vi "ALTS-2015 Robot Controller Loop.vi"(8 "error in (no error)":errorcluster) -> (0 "error out":errorcluster)   [LabVIEW 2013]
uses:
  Controls/ALTS-2015 Serial Details.ctl
  Controls/ALTS-2015 Robot Tasks.ctl
  Controls/ALTS-2015 Station Cluster.ctl
  Controls/ALTS-2015 Serial DB Details.ctl
  Robot Controller Queue/ALTS-2015 Robot Cotroller Options.ctl
  Controls/ALTS-2015 Auto Program States.ctl
  OPC Engine/Controls/ALTS-2015 OPC Read Registers.ctl
  OPC Engine/Controls/ALTS-2015 OPC Read Global Options.ctl
  Controls/ALTS-2015 Status Message Options.ctl
  Controls/ALTS-2015 Station Details.ctl
  Controls/ALTS-2015 Status Ring Indicator.ctl
  Controls/ALTS-2015 Robot Actions.ctl
  Controls/ALTS-2015 LV2GBL Station Info Options.ctl
  Controls/ALTS-2015 Robot FIFO Queue Options.ctl
  OPC Engine/Controls/ALTS-2015 OPC Write Registers.ctl
  OPC Engine/Controls/ALTS-2015 OPC Write Global Options.ctl
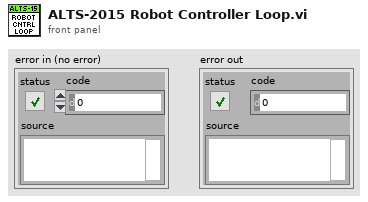
[diagram p1: front panel]
types:
  T1 = typedef "ALTS-2015 Robot Cotroller Options.ctl" = enum16{"Init", "Enqueue State", "Enqueue State in Opposite End", "Dequeue State", "Exit"}
  T2 = typedef "ALTS-2015 Auto Program States.ctl" = enum16{"<------ Robot Handler States ------>", "Wait for Robot Availability", "Check Last Task by Robot", "Wait & Read Task from Queue", "Write New Task Details to Robot", "Write Task Available for Robot", "Check Robot for Unavailbilty", "Write Task Unavailable for Robot", "<------------ Other ------------>", "Error", "Exit"}
  T3 = typedef "ALTS-2015 Serial Details.ctl" = cluster{"Robot Task":T4, "Serial No":string, "New Serial?":bool, "Station # Unload":T5, "Last Test Result":bool, "Rerun?":bool, "Station # Rerun":T5, "Invalid Serial?":bool, "Serial Details":T6}
  T4 = typedef "ALTS-2015 Robot Tasks.ctl" = enum16{"Load", "Unload", "Rerun", "Invalid Serial"}
  T5 = typedef "ALTS-2015 Station Cluster.ctl" = enum16{"Station 1", "Station 2", "Station 3", "Station 4"}
  T6 = typedef "ALTS-2015 Serial DB Details.ctl" = cluster{"Adapter Plate Size":i32, "Air Leak Test Type ":i32, "Displacement Size":i32, "Flange Size":i32, "Height":i32, "Load Decision":i32, "Cart Insert":i32}
  T7 = cluster{"Serial Details":T3, "Last Robot Task":T4, "Last Robot Task Out Station #":T5, "Robot Task broadcased?":bool}
  T8 = typedef "ALTS-2015 OPC Read Global Options.ctl" = enum16{"Init", "Write Value", "Write Array", "Read Value", "Read Array", "Read All"}
  T9 = typedef "ALTS-2015 OPC Read Registers.ctl" = enum16{"Robot_Available", "Start_Test", "Stop_Test", "Scan_Trigger", "Station_No_Start_Stop_Test"}
  T10 = typedef "ALTS-2015 Status Message Options.ctl" = enum16{"Initializing...", "Enter User Login...", "Valid Serial Number...", "Invalid Serial Number...", "Start Tag Received...", "Stop Tag Received...", "UUT Clamped...", "UUT not Clamped...", "Test Running...", "Test Complete...", "Task is assigned to robot...", "Robot is working on the task...", "Robot is ready for next task...", "Writing Result to DB...", "Idle...", "Exiting..."}
  T11 = typedef "ALTS-2015 LV2GBL Station Info Options.ctl" = enum16{"Init", "Read", "Read All", "Write Sensor ID", "Write  Work Order", "Write Serial Number", "Write Test Data", "Write Station Status", "Write Station Occupancy", "Write Station Test Type", "Write Rerun", "Write Load Decision", "Write Robot Action", "Clear All", "Clear Test Result"}
  T12 = typedef "ALTS-2015 Robot Actions.ctl" = enum16{"Loading...", "Unloading...", "Reruning...", "No Action"}
  T13 = typedef "ALTS-2015 Station Details.ctl" = cluster{"Station Number":string, "Work Order Number":string, "Sensor Name":string, "Pressure (PSI)":string, "Flow (SCCM)":string, "Test Time ":string, "Test Result":string, "Serial Number":string, "Station Status":T14, "SW assigned UUT":bool, "Rerun Count":i32, "Test Type":i32, "Load Decision":i32, "Robot Action":T12}
  T14 = typedef "ALTS-2015 Status Ring Indicator.ctl" = u16
  T15 = typedef "ALTS-2015 Robot FIFO Queue Options.ctl" = enum16{"Init", "Enqueue", "Dequeue", "Get Queue Elements", "Flush", "Destroy"}
  T16 = typedef "ALTS-2015 OPC Write Global Options.ctl" = enum16{"Init", "Write Value", "Write Array", "Read Value", "Read Array", "Read All"}
  T17 = typedef "ALTS-2015 OPC Write Registers.ctl" = enum16{"Task_Available_for_Robot", "New_Serial", "Serial_Adapter_Size", "Serial_Displacement_Size", "Serial_Flange_Size", "Serial_Height", "Serial_LoadDecision", "Serial_CartInsert", "Test_Result", "Station_Number", "Rerun", "Invalid_SNo", "PC_ACK_Read_Tags"}
  T18 = enum16{"Init", "Set - DB Loop", "Set - Robot Loop", "Get"}
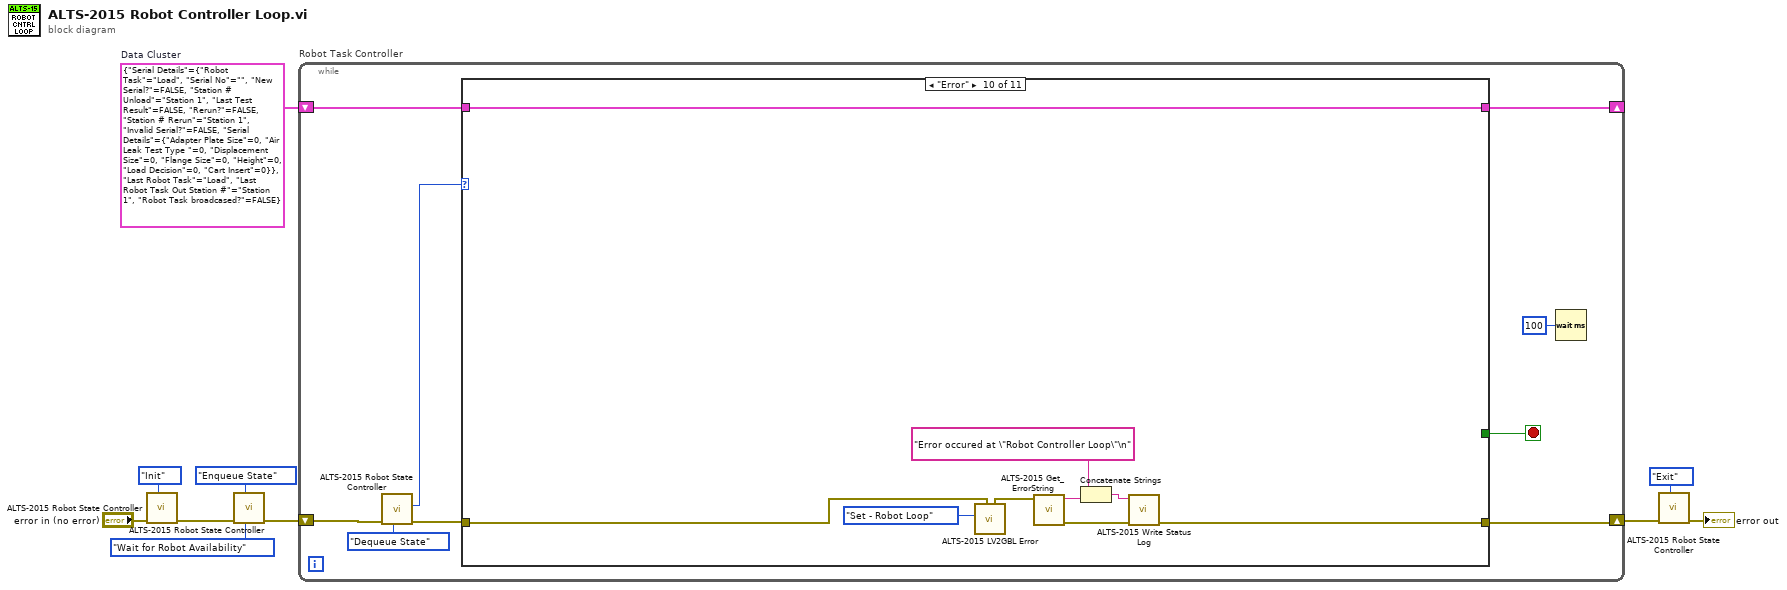
[diagram p0: block diagram]
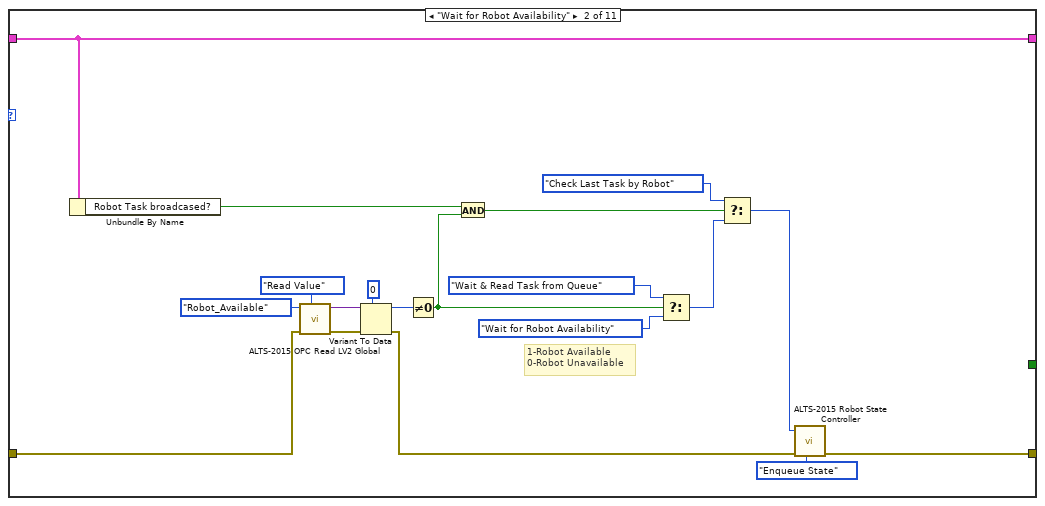
[diagram p3: hidden frame]
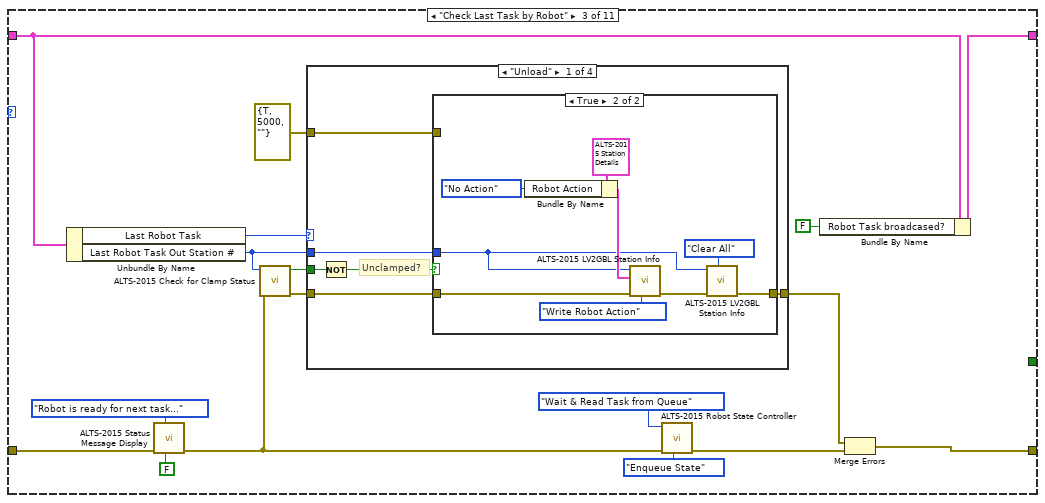
[diagram p4: hidden frame]
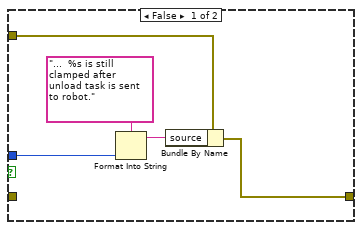
[diagram p5: hidden frame]
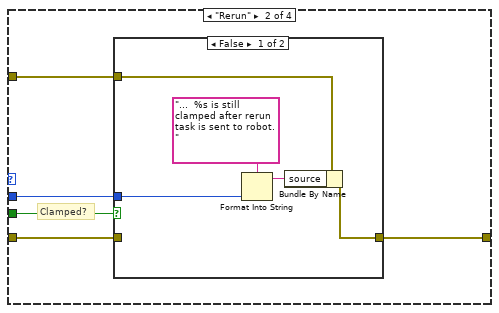
[diagram p6: hidden frame]
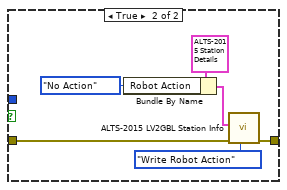
[diagram p7: hidden frame]
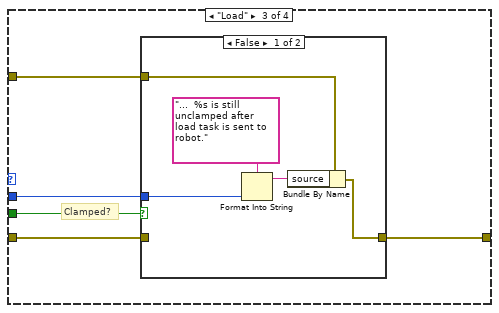
[diagram p8: hidden frame]
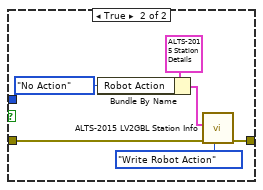
[diagram p9: hidden frame]
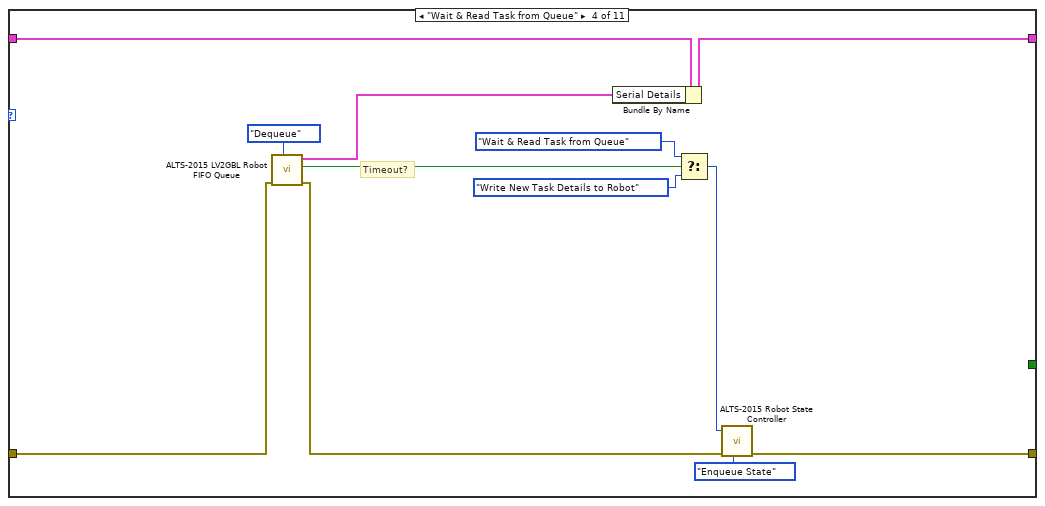
[diagram p11: hidden frame]
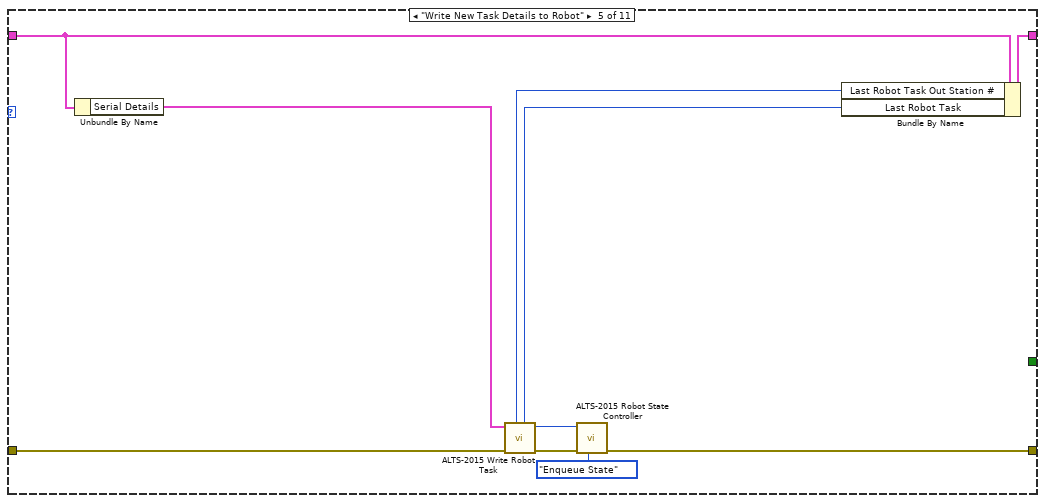
[diagram p12: hidden frame]
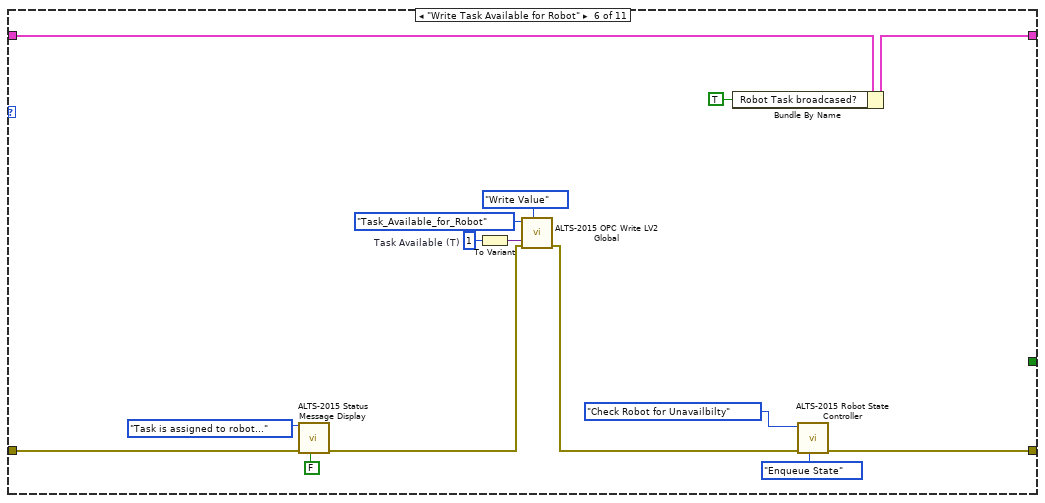
[diagram p13: hidden frame]
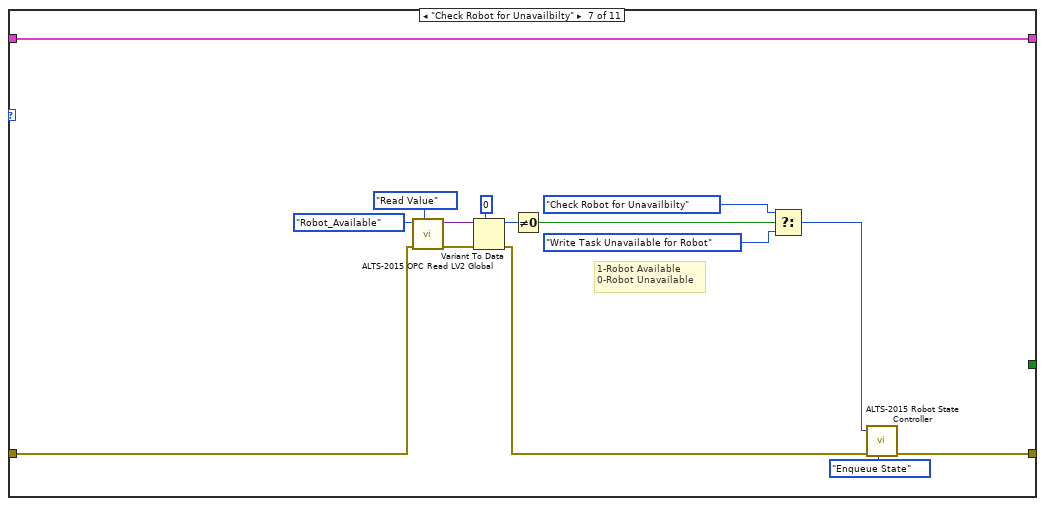
[diagram p14: hidden frame]
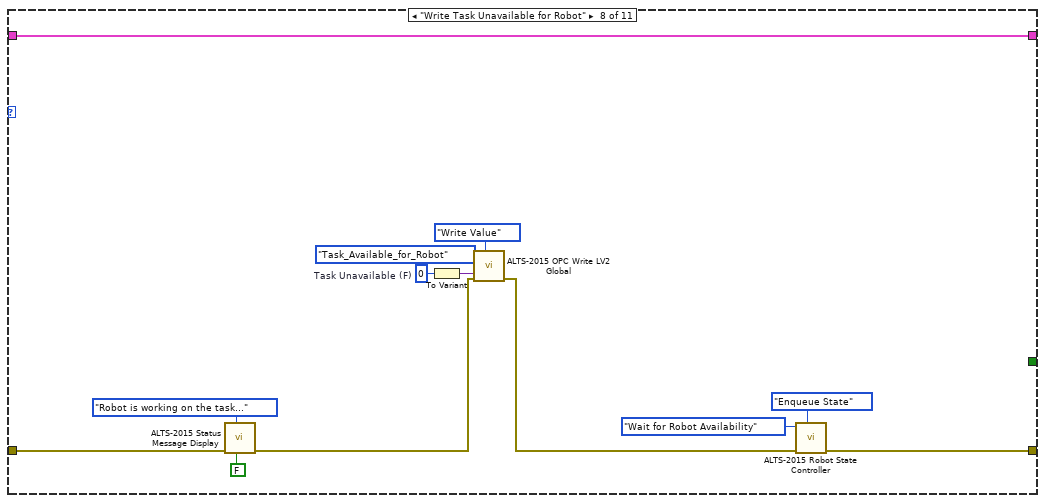
[diagram p15: hidden frame]
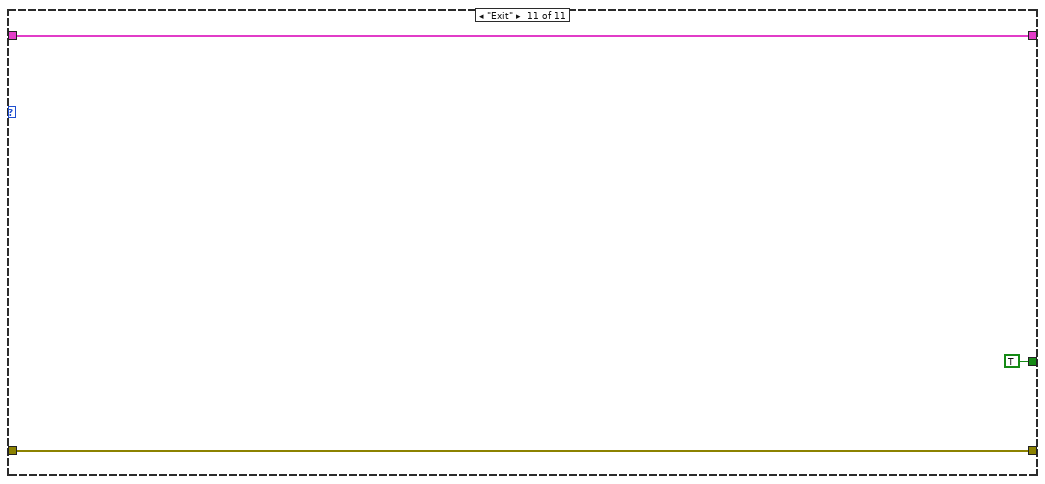
[diagram p17: hidden frame]
diagram:
  w9 = T7 {"Serial Details"={"Robot Task"=enum."Load", "Serial No"="", "New Serial?"=FALSE, "Station # Unload"=enum."Station 1", "Last Test Result"=FALSE, "Rerun?"=FALSE, "Station # Rerun"=enum."Station 1", "Invalid Serial?"=FALSE, "Serial Details"={"Adapter Plate Size"=0, "Air Leak Test Type "=0, "Displacement Size"=0, "Flange Size"=0, "Height"=0, "Load Decision"=0, "Cart Insert"=0}}, "Last Robot Task"=enum."Load", "Last Robot Task Out Station #"=enum."Station 1", "Robot Task broadcased?"=FALSE}  # Data Cluster
  n1 = call "ALTS-2015 Robot State Controller.vi"("Option"=ALTS-2015_Robot_Cotroller_Options."Init", "error in"="error in (no error)") -> ("error out"=w7:errorcluster)  [unwired: 8 in, 1 out]
  n2 = call "ALTS-2015 Robot State Controller.vi"("Option"=ALTS-2015_Robot_Cotroller_Options."Enqueue State", "error in"=w7, "Enqueue State"=ALTS-2015_Auto_Program_States."Wait for Robot Availability") -> ("error out"=w5:errorcluster)  [unwired: 7 in, 1 out]
  n3 = while "Robot Task Controller" {
    shift-right: [w11] -> w10
    shift-left: w5 -> [w15]
    shift-right: [w17] -> _
    shift-left: w9 -> [w18]
    stop <- w16 stop-if-true
    n4 = call "ALTS-2015 Robot State Controller.vi"("Option"=ALTS-2015_Robot_Cotroller_Options."Dequeue State", "error in"=w15) -> ("error out"=w14:errorcluster, "Dequeued State"=w13:T2)  [unwired: 8 in]
    n5 = case shown="\"Error\"" w13 {
      tunnel: [w20 w30 w43 w113 w128 w141 w150 w169 w176 w185 w188] -> w11
      tunnel: w14 -> [w20 w32 w44 w118 w132 w135 w156 w164 w176 w179 w188]
      tunnel: w18 -> [w21 w27 w55 w117 w131 w143 w153 w171 w177 w186 w189]
      tunnel: [w21 w27 w50 w116 w125 w138 w153 w171 w177 w186 w189] -> w17
      tunnel: [_ _ _ _ _ _ _ _ _ _ TRUE] -> w16
      frame "<------ Robot Handler States ------>" {
      }
      frame "Wait for Robot Availability" {
        # "1-Robot Available\n0-Robot Unavailable"
        n6 = Unbundle By Name(w27) -> ("Robot Task broadcased?"=w25:bool)
        n7 = call "ALTS-2015 OPC Read LV2 Global.vi"("Options"=ALTS-2015_OPC_Read_Global_Options."Read Value", "error in (no error)"=w32, "OPC Read Register"=ALTS-2015_OPC_Read_Registers."Robot_Available") -> ("error out"=w38:errorcluster, "OPC Read Reigter Value"=w39:variant)  [unwired: 6 in, 1 out]
        n8 = Variant To Data(error in=w38, type=0, Variant=w39) -> (data=w35:i32, error out=w31:errorcluster)
        n9 = Not Equal To 0?(x=w35) -> (x != 0?=w22:bool)
        n10 = And(x=w25, y=w22) -> (x .and. y?=w23:bool)
        n11 = Select(t=ALTS-2015_Auto_Program_States."Wait & Read Task from Queue", s=w22, f=ALTS-2015_Auto_Program_States."Wait for Robot Availability") -> (s? t:f=w29:T2)
        n12 = Select(t=ALTS-2015_Auto_Program_States."Check Last Task by Robot", s=w23, f=w29) -> (s? t:f=w26:T2)
        n13 = call "ALTS-2015 Robot State Controller.vi"("Option"=ALTS-2015_Robot_Cotroller_Options."Enqueue State", "error in"=w31, "Enqueue State"=w26) -> ("error out"=w30:errorcluster)  [unwired: 7 in, 1 out]
      }
      frame "Check Last Task by Robot" {
        n14 = Unbundle By Name(w55) -> ("Last Robot Task"=w51:T4, "Last Robot Task Out Station #"=w54:T5)
        n15 = call "ALTS-2015 Status Message Display.vi"("Station Message?"=FALSE, "Status Message Options"=ALTS-2015_Status_Message_Options."Robot is ready for next task...", "error in (no error)"=w44) -> ("error out"=w41:errorcluster)  [unwired: 7 in, 1 out]
        n16 = call "ALTS-2015 Check for Clamp Status .vi"("error in (no error)"=w41, "Station Cluster"=w54) -> ("error out"=w53:errorcluster, "Clamp?"=w52:bool)  [unwired: 8 in]
        n17 = case shown="\"Unload\"" w51 {
          tunnel: w54 -> [w63 w82 w98 _]
          tunnel: [w62 w81 w97 w110] -> w42
          tunnel: w53 -> [w61 w80 w96 w110]
          tunnel: w52 -> [w60 w79 w95 _]
          tunnel: errorcluster {"status"=TRUE, "code"=5000, "source"=""} ("error constant") -> [w58 w78 w94 _]
          frame "Unload" {
            # "Unclamped?"
            n18 = Not(x=w60) -> (.not. x?=w59:bool)
            n19 = case shown="True" w59 {
              tunnel: w63 -> [w68 w69]
              tunnel: w61 -> [_ w77]
              tunnel: [w66 w70] -> w62
              tunnel: w58 -> [w67 _]
              frame False {
                n20 = Format Into String(format string="...  %s is still clamped after unload task is sent to robot." ("Status Input"), w68) -> (resulting string=w64:string)  [unwired: 2 in, 1 out]
                n21 = Bundle By Name(cluster=w67, "source"=w64) -> (w66:errorcluster)
              }
              frame True {
                n22 = Bundle By Name(cluster=T13 {"Station Number"="", "Work Order Number"="", "Sensor Name"="", "Pressure (PSI)"="", "Flow (SCCM)"="", "Test Time "="", "Test Result"="", "Serial Number"="", "Station Status"=0, "SW assigned UUT"=FALSE, "Rerun Count"=0, "Test Type"=0, "Load Decision"=0, "Robot Action"=enum."Loading..."} ("Station"), "Robot Action"=ALTS-2015_Robot_Actions."No Action") -> (w75:T13)
                n23 = call "ALTS-2015 LV2GBL Station Info.vi"("Options"=ALTS-2015_LV2GBL_Station_Info_Options."Write Robot Action", "error in"=w77, "Station"=w75, "Station Cluster"=w69) -> ("error out"=w71:errorcluster)  [unwired: 5 in, 2 out]
                n24 = call "ALTS-2015 LV2GBL Station Info.vi"("Options"=ALTS-2015_LV2GBL_Station_Info_Options."Clear All", "error in"=w71, "Station Cluster"=w69) -> ("error out"=w70:errorcluster)  [unwired: 6 in, 2 out]
              }
            }
          }
          frame "Rerun" {
            # "Clamped?"
            n25 = case shown="False" w79 {
              tunnel: w82 -> [w87 _]
              tunnel: w80 -> [_ w90]
              tunnel: [w86 w89] -> w81
              tunnel: w78 -> [w84 _]
              frame False {
                n26 = Format Into String(format string="...  %s is still clamped after rerun task is sent to robot." ("Status Input"), w87) -> (resulting string=w83:string)  [unwired: 2 in, 1 out]
                n27 = Bundle By Name(cluster=w84, "source"=w83) -> (w86:errorcluster)
              }
              frame True {
                n28 = Bundle By Name(cluster=T13 {"Station Number"="", "Work Order Number"="", "Sensor Name"="", "Pressure (PSI)"="", "Flow (SCCM)"="", "Test Time "="", "Test Result"="", "Serial Number"="", "Station Status"=0, "SW assigned UUT"=FALSE, "Rerun Count"=0, "Test Type"=0, "Load Decision"=0, "Robot Action"=enum."Loading..."} ("Station"), "Robot Action"=ALTS-2015_Robot_Actions."No Action") -> (w92:T13)
                n29 = call "ALTS-2015 LV2GBL Station Info.vi"("Options"=ALTS-2015_LV2GBL_Station_Info_Options."Write Robot Action", "error in"=w90, "Station"=w92) -> ("error out"=w89:errorcluster)  [unwired: 6 in, 2 out]
              }
            }
          }
          frame "Load" {
            # "Clamped?"
            n30 = case shown="False" w95 {
              tunnel: w98 -> [w103 _]
              tunnel: w96 -> [_ w106]
              tunnel: [w100 w105] -> w97
              tunnel: w94 -> [w102 _]
              frame False {
                n31 = Format Into String(format string="...  %s is still unclamped after load task is sent to robot." ("Status Input"), w103) -> (resulting string=w99:string)  [unwired: 2 in, 1 out]
                n32 = Bundle By Name(cluster=w102, "source"=w99) -> (w100:errorcluster)
              }
              frame True {
                n33 = Bundle By Name(cluster=T13 {"Station Number"="", "Work Order Number"="", "Sensor Name"="", "Pressure (PSI)"="", "Flow (SCCM)"="", "Test Time "="", "Test Result"="", "Serial Number"="", "Station Status"=0, "SW assigned UUT"=FALSE, "Rerun Count"=0, "Test Type"=0, "Load Decision"=0, "Robot Action"=enum."Loading..."} ("Station"), "Robot Action"=ALTS-2015_Robot_Actions."No Action") -> (w108:T13)
                n34 = call "ALTS-2015 LV2GBL Station Info.vi"("Options"=ALTS-2015_LV2GBL_Station_Info_Options."Write Robot Action", "error in"=w106, "Station"=w108) -> ("error out"=w105:errorcluster)  [unwired: 6 in, 2 out]
              }
            }
          }
          frame Default {
          }
        }
        n35 = call "ALTS-2015 Robot State Controller.vi"("Option"=ALTS-2015_Robot_Cotroller_Options."Enqueue State", "error in"=w41, "Enqueue State"=ALTS-2015_Auto_Program_States."Wait & Read Task from Queue") -> ("error out"=w57:errorcluster)  [unwired: 7 in, 1 out]
        n36 = Bundle By Name(cluster=w55, "Robot Task broadcased?"=FALSE) -> (w50:T7)
        n37 = Merge Errors(w42, w57) -> (w43:errorcluster)
      }
      frame "Wait & Read Task from Queue" {
        # "Timeout?"
        n38 = call "ALTS-2015 LV2GBL Robot FIFO Queue.vi"("Options"=ALTS-2015_Robot_FIFO_Queue_Options."Dequeue" ("Enum"), "error in (no error)"=w118) -> ("error out"=w114:errorcluster, "timed out?"=w121:bool, "Task Details Out"=w115:T3)  [unwired: 5 in, 2 out]
        n39 = Bundle By Name(cluster=w117, "Serial Details"=w115) -> (w116:T7)
        n40 = Select(t=ALTS-2015_Auto_Program_States."Wait & Read Task from Queue", s=w121, f=ALTS-2015_Auto_Program_States."Write New Task Details to Robot") -> (s? t:f=w112:T2)
        n41 = call "ALTS-2015 Robot State Controller.vi"("Option"=ALTS-2015_Robot_Cotroller_Options."Enqueue State", "error in"=w114, "Enqueue State"=w112) -> ("error out"=w113:errorcluster)  [unwired: 7 in, 1 out]
      }
      frame "Write New Task Details to Robot" {
        n42 = Unbundle By Name(w131) -> ("Serial Details"=w130:T3)
        n43 = call "ALTS-2015 Write Robot Task.vi"("error in (no error)"=w132, "Task Details"=w130) -> ("error out"=w129:errorcluster, "Next State to Execute"=w127:T2, "Last Robot Task"=w124:T4, "Last Robot Task Out Station #"=w123:T5)  [unwired: 6 in]
        n44 = call "ALTS-2015 Robot State Controller.vi"("Option"=ALTS-2015_Robot_Cotroller_Options."Enqueue State", "error in"=w129, "Enqueue State"=w127) -> ("error out"=w128:errorcluster)  [unwired: 7 in, 1 out]
        n45 = Bundle By Name(cluster=w131, "Last Robot Task Out Station #"=w123, "Last Robot Task"=w124) -> (w125:T7)
      }
      frame "Write Task Available for Robot" {
        w147 = 1  # Task Available (T)
        n46 = call "ALTS-2015 Status Message Display.vi"("Station Message?"=FALSE, "Status Message Options"=ALTS-2015_Status_Message_Options."Task is assigned to robot...", "error in (no error)"=w135) -> ("error out"=w134:errorcluster)  [unwired: 7 in, 1 out]
        n47 = To Variant(anything=w147) -> (Variant=w146:variant)
        n48 = call "ALTS-2015 OPC Write LV2 Global.vi"("Options"=ALTS-2015_OPC_Write_Global_Options."Write Value", "error in (no error)"=w134, "OPC value"=w146, "OPC Write Register"=ALTS-2015_OPC_Write_Registers."Task_Available_for_Robot") -> ("error out"=w142:errorcluster)  [unwired: 5 in, 2 out]
        n49 = Bundle By Name(cluster=w143, "Robot Task broadcased?"=TRUE) -> (w138:T7)
        n50 = call "ALTS-2015 Robot State Controller.vi"("Option"=ALTS-2015_Robot_Cotroller_Options."Enqueue State", "error in"=w142, "Enqueue State"=ALTS-2015_Auto_Program_States."Check Robot for Unavailbilty") -> ("error out"=w141:errorcluster)  [unwired: 7 in, 1 out]
      }
      frame "Check Robot for Unavailbilty" {
        # "1-Robot Available\n0-Robot Unavailable"
        n51 = call "ALTS-2015 OPC Read LV2 Global.vi"("Options"=ALTS-2015_OPC_Read_Global_Options."Read Value", "error in (no error)"=w156, "OPC Read Register"=ALTS-2015_OPC_Read_Registers."Robot_Available") -> ("error out"=w160:errorcluster, "OPC Read Reigter Value"=w161:variant)  [unwired: 6 in, 1 out]
        n52 = Variant To Data(error in=w160, type=0, Variant=w161) -> (data=w157:i32, error out=w151:errorcluster)
        n53 = Not Equal To 0?(x=w157) -> (x != 0?=w152:bool)
        n54 = Select(t=ALTS-2015_Auto_Program_States."Check Robot for Unavailbilty", s=w152, f=ALTS-2015_Auto_Program_States."Write Task Unavailable for Robot") -> (s? t:f=w149:T2)
        n55 = call "ALTS-2015 Robot State Controller.vi"("Option"=ALTS-2015_Robot_Cotroller_Options."Enqueue State", "error in"=w151, "Enqueue State"=w149) -> ("error out"=w150:errorcluster)  [unwired: 7 in, 1 out]
      }
      frame "Write Task Unavailable for Robot" {
        w175 = 0  # Task Unavailable (F)
        n56 = call "ALTS-2015 Status Message Display.vi"("Station Message?"=FALSE, "Status Message Options"=ALTS-2015_Status_Message_Options."Robot is working on the task...", "error in (no error)"=w164) -> ("error out"=w163:errorcluster)  [unwired: 7 in, 1 out]
        n57 = To Variant(anything=w175) -> (Variant=w174:variant)
        n58 = call "ALTS-2015 OPC Write LV2 Global.vi"("Options"=ALTS-2015_OPC_Write_Global_Options."Write Value", "error in (no error)"=w163, "OPC value"=w174, "OPC Write Register"=ALTS-2015_OPC_Write_Registers."Task_Available_for_Robot") -> ("error out"=w170:errorcluster)  [unwired: 5 in, 2 out]
        n59 = call "ALTS-2015 Robot State Controller.vi"("Option"=ALTS-2015_Robot_Cotroller_Options."Enqueue State", "error in"=w170, "Enqueue State"=ALTS-2015_Auto_Program_States."Wait for Robot Availability") -> ("error out"=w169:errorcluster)  [unwired: 7 in, 1 out]
      }
      frame "<------------ Other ------------>" {
      }
      frame "Error" {
        n60 = call "ALTS-2015 LV2GBL Error.vi"("error in - Robot Loop"=w179, "Operation"=T18."Set - Robot Loop") -> ("error out  - Robot Loop"=w178:errorcluster)  [unwired: 8 in, 1 out]
        n61 = call "ALTS-2015 Get_ErrorString.vi"("Incoming Error"=w178) -> ("error out"=w184:errorcluster, "Message"=w183:string)  [unwired: 9 in]
        n62 = Concatenate Strings("Error occured at \"Robot Controller Loop\"\n" ("string"), w183) -> (w182:string)
        n63 = call "ALTS-2015 Write Status Log.vi"("error in (no error)"=w184, "Status Input"=w182) -> ("error out"=w185:errorcluster)  [unwired: 9 in]
      }
      frame "Exit" {
      }
    }
    n64 = Wait (ms)(milliseconds to wait=u32 100) -> ()  [unwired: 1 out]
  }
  n65 = call "ALTS-2015 Robot State Controller.vi"("Option"=ALTS-2015_Robot_Cotroller_Options."Exit", "error in"=w10) -> ("error out"=→"error out":errorcluster)  [unwired: 8 in, 1 out]
